vi "SRV_Check Prdouct found.vi"(8 "error in (no error)":errorcluster, 10 "Prd Name":string, 11 "Refnum in":T1) -> (0 "error out":errorcluster, 2 "Found":bool, 3 "Refnum out":T1)   [LabVIEW 2015]
uses:
  <vilib>/addons/database/Connection.llb/Conn ObjectReference.ctl
  <userlib>/user.lib/origin_lib_main/db_interface/DB Operations Enum.ctl
  <vilib>/addons/database/_DB Variant To Data/Database Variant To Data.xnode
  <userlib>/user.lib/origin_lib_main/db_interface/DB Interface.lvlib
  <vilib>/addons/database/NI_Database_API.lvlib
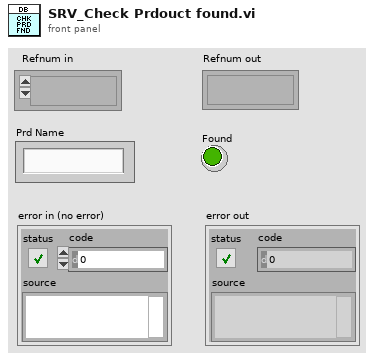
[diagram p1: front panel]
types:
  T1 = typedef "NI_Database_API.lvlib/Conn ObjectReference.ctl" = refnum<k1>
  T2 = typedef "DB Interface.lvlib/DB Operations Enum.ctl" = enum16{"Select", "Update", "Insert", "Delete", "Fetch SQL Query", "Execute SQL Query", "Drop Table", "List Tables"}
  T3 = enum32{"Bad", "Idle", "Run top level", "Running"}
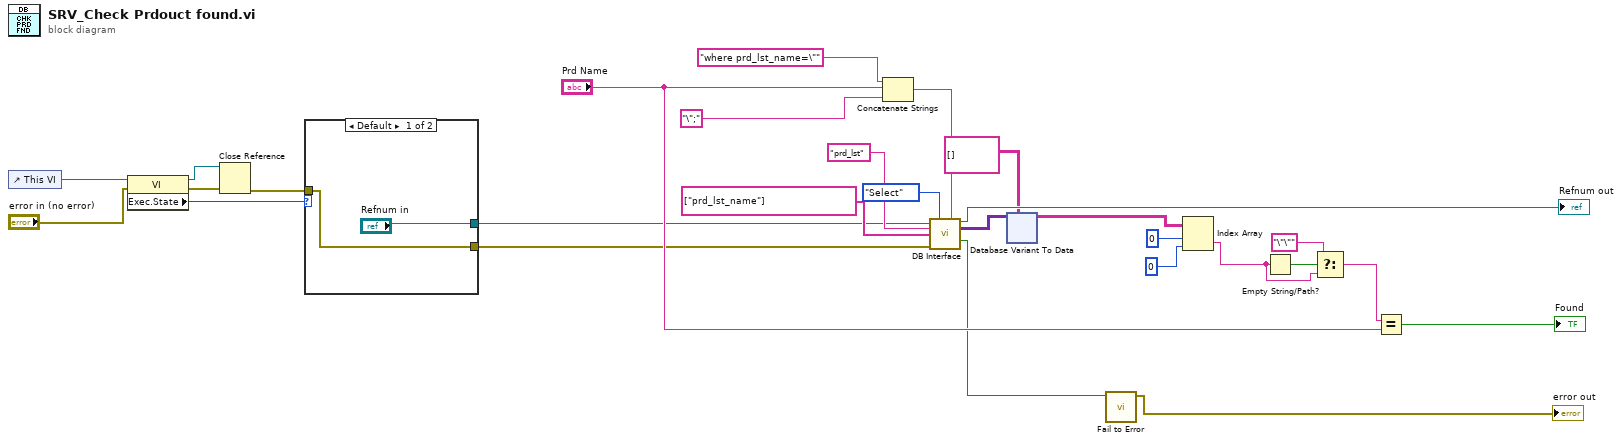
[diagram p0: block diagram]
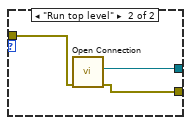
[diagram p2: hidden frame]
diagram:
  n1 = control-ref of="This VI"() -> (w11:refnum<vi>)
  n2 = property class="VI"(reference=w11, error in="error in (no error)") -> (reference out=w9:refnum<vi>, error out=w8:errorcluster, "Exec.State"=w10:T3)
  n3 = Close Reference(reference=w9, error in (no error)=w8) -> (error out=w6:errorcluster)
  n4 = case shown="Default" w10 {
    tunnel: w6 -> [w29 w32]
    tunnel: ["Refnum in" w33] -> w5
    tunnel: [w29 w31] -> w4
    frame Default {
    }
    frame "Run top level" {
      n5 = call "Open Connection.vi"("error in (no error)"=w32) -> ("error out"=w31:errorcluster, "connection reference"=w33:T1)  [unwired: 8 in, 1 out]
    }
  }
  n6 = Concatenate Strings("where prd_lst_name=\"" ("condition"), "Prd Name", "\";" ("string")) -> (w18:string)
  n7 = call <userlib>:"DB Interface.vi"("DB Ref In"=w5, "Operation"=DB_Operations_Enum."Select", "condition"=w18, "DB Table"="prd_lst" ("table"), "DB columns"=string[] ["prd_lst_name"] ("columns"), "error in (no error)"=w4) -> ("DB Ref Out"=→"Refnum out":T1, "data Out"=w22:variant[][], "Sucess ?"=w2:bool)  [unwired: 6 in, 1 out]
  n8 = xnode "Database Variant To Data"("database variant"=w22, "type"=string[][] []) -> ("data"=w26:string[][])  [unwired: 1 in, 1 out]
  n9 = call "Fail to Error.vi"("Sucess ?"=w2) -> ("error out"=→"error out":errorcluster)  [unwired: 10 in]
  n10 = Index Array(array=w26, index (row)=0, index (col)=0 ("disabled index (col)")) -> (element=w15:string)
  n11 = Empty String/Path?(string/path=w15) -> (empty?=w16:bool)
  n12 = Select(t="\"\"", s=w16, f=w15) -> (s? t:f=w14:string)
  n13 = Equal?(x=w14, y="Prd Name") -> (x = y?=→"Found":bool)
